vi "HandleGetState.vi"(0 "reference in":refnum<class "Device.lvclass">, 5 "message in":T1, 11 "error in (no error)":errorcluster) -> (4 "reference out":refnum<class "Device.lvclass">, 15 "error out":errorcluster)   [LabVIEW 2019]
uses:
  Device.lvclass
  MessageInterface_class/Message.ctl
  Proccess_class/Proccess.lvclass
  MessageInterface_class/MessageInterface.lvclass
  D:/H4000/src/Proccess_class/Proccess.lvclass
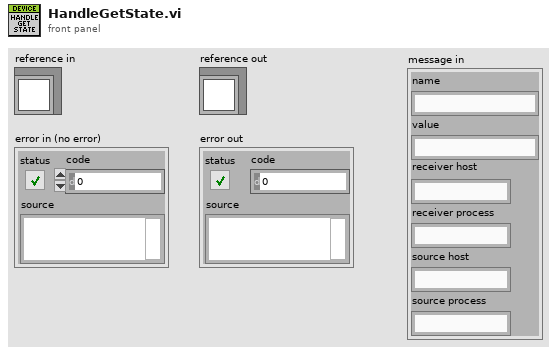
[diagram p1: front panel]
types:
  T1 = typedef "MessageInterface.lvclass/Message.ctl" = cluster{"name":string, "value":string, "receiver host":string, "receiver process":string, "source host":string, "source process":string}
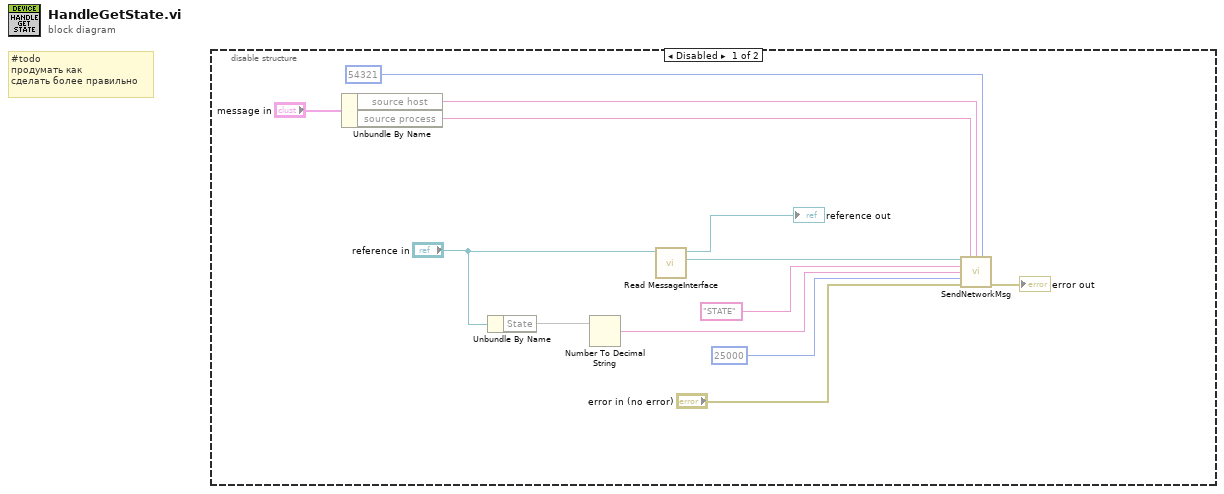
[diagram p0: block diagram]
diagram:
  # "#todo\nпродумать как \nсделать более правильно"
  n1 = disable-structure shown="Disabled" {
    frame Disabled {
      n2 = Unbundle By Name("message in") -> ("source host"=w10:string, "source process"=w9:string)
      n3 = Unbundle By Name("reference in") -> ("State"=w7)
      n4 = Number To Decimal String(number=w7) -> (decimal integer string=w6:string)  [unwired: 1 in]
      n5 = call "Read MessageInterface.vi"("Proccess in"="reference in") -> ("MessageInterface"=w2:refnum<class "MessageInterface.lvclass">, "Proccess out"=→"reference out":refnum<class "Device.lvclass">)  [unwired: 9 in]
      n6 = call-dynamic "SendNetworkMsg.vi"("reference in"=w2, "receiver process"=w9, "receiver host"=w10, "receiver port (0)"=u16 54321 ("UDP port"), "name"="STATE", "value"=w6, "timeout (25000 ms)"=25000, "error in (no error)"="error in (no error)") -> ("error out"=→"error out":errorcluster)  [unwired: 5 in, 2 out]
    }
    frame Enabled {
    }
  }
